vi "Write Multi-D.vi"(7 "D Array":i16[](array[numeric]), 8 "Error In":errorcluster, 9 "Length":u16, 10 "Position (U32)":u32, 11 "connection ID":refnum<k5>) -> (0 "Error Out":errorcluster, 3 "connection ID out":refnum<k5>)   [LabVIEW 2019, in "FX5U SLMP Binary.lvlib"]
uses:
  FX5U SLMP Binary.lvlib
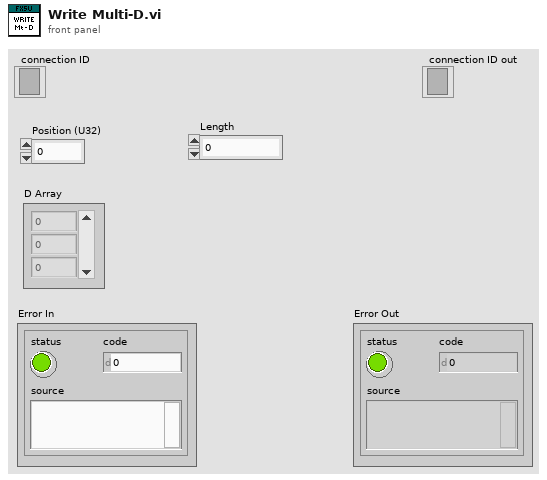
[diagram p1: front panel]
types:
  T1 = enum16{"big-endian, network order", "native, host order", "little-endian"}
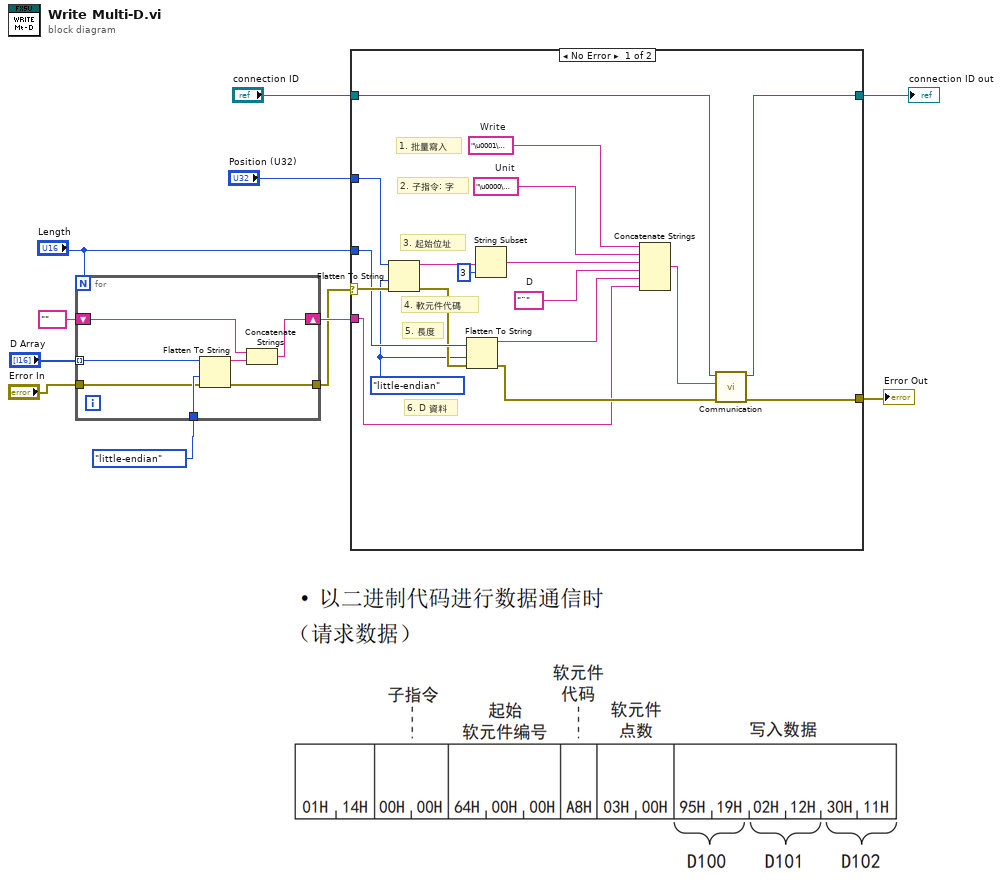
[diagram p0: block diagram]
diagram:
  n1 = for {
    N: "Length" -> [_]
    tunnel: "D Array" -> [w18] mode=indexing
    shift-right: [w16] -> w3
    shift-left: "" -> [w15]
    tunnel: T1."little-endian" ("byte order (0:big-endian, network order)") -> [w14]
    tunnel: "Error In" -> [w13]
    tunnel: [w12] -> w1
    n2 = Flatten To String(anything=w18, byte order (0:big-endian, network order)=w14, error in (no error)=w13) -> (data string=w17:string, error out=w12:errorcluster)  [unwired: 1 in, 1 out]
    n3 = Concatenate Strings(w15, w17) -> (w16:string)
  }
  n4 = case shown="No Error" w1 {
    selector: w1 -> [w35 w38]
    tunnel: "Position (U32)" -> [w36 _]
    tunnel: [w30 w38] -> w10
    tunnel: "connection ID" -> [w29 w37]
    tunnel: [w28 w37] -> w8
    tunnel: "Length" -> [w24 _]
    tunnel: w3 -> [w20 _]
    frame No Error {
      w19 = T1."little-endian" ("byte order (0:big-endian, network order)")
      w25 = "¨"  # D
      w33 = "\u0000\u0000"  # Unit
      w34 = "\u0001\u0014"  # Write
      # "6. D 資料"
      # "5. 長度"
      # "4. 軟元件代碼"
      # "3. 起始位址"
      # "2. 子指令: 字"
      # "1. 批量寫入"
      n5 = Flatten To String(anything=w36, byte order (0:big-endian, network order)=w19, error in (no error)=w35) -> (data string=w32:string, error out=w23:errorcluster)  [unwired: 1 in, 1 out]
      n6 = Flatten To String(anything=w24, byte order (0:big-endian, network order)=w19, error in (no error)=w23) -> (data string=w22:string, error out=w21:errorcluster)  [unwired: 1 in, 1 out]
      n7 = String Subset(string=w32, length (rest)=3 ("length (rest)")) -> (substring=w26:string)  [unwired: 1 in]
      n8 = Concatenate Strings(w34, w33, w26, w25, w22, w20) -> (w27:string)
      n9 = call "Communication.vi"("Error In"=w21, "Command"=w27, "connection ID"=w29) -> ("Error Out"=w30:errorcluster, "connection ID out"=w28:refnum<k5>)  [unwired: 6 in, 1 out]
    }
    frame Error {
    }
  }
  "Error Out" <- w10
  "connection ID out" <- w8
